vi "I2C_read.vi"(10 "错误输入（无错误）":errorcluster) -> (0 "readSucess":bool, 1 "buf":u8[](array[numeric]), 2 "Led":string, 3 "错误输出":errorcluster)   [LabVIEW 2017]
uses:
  jtool.dll
panel:
  out "reg_addr":u32
  out "slave_addr":u8
  out "init":string
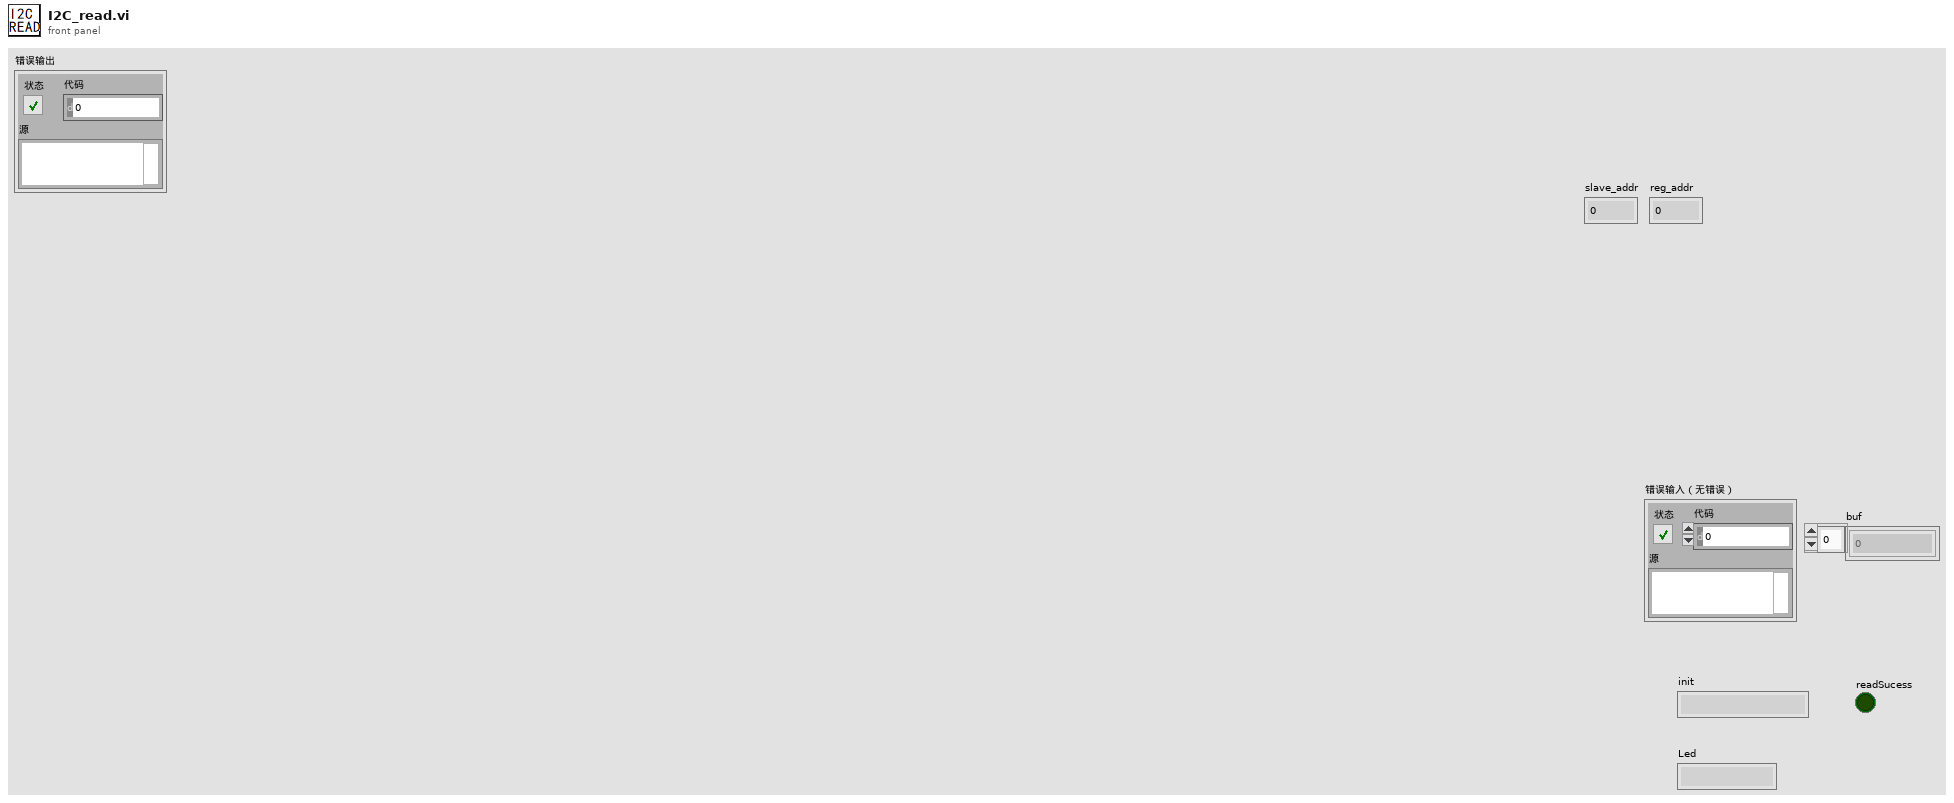
[diagram p1: front panel]
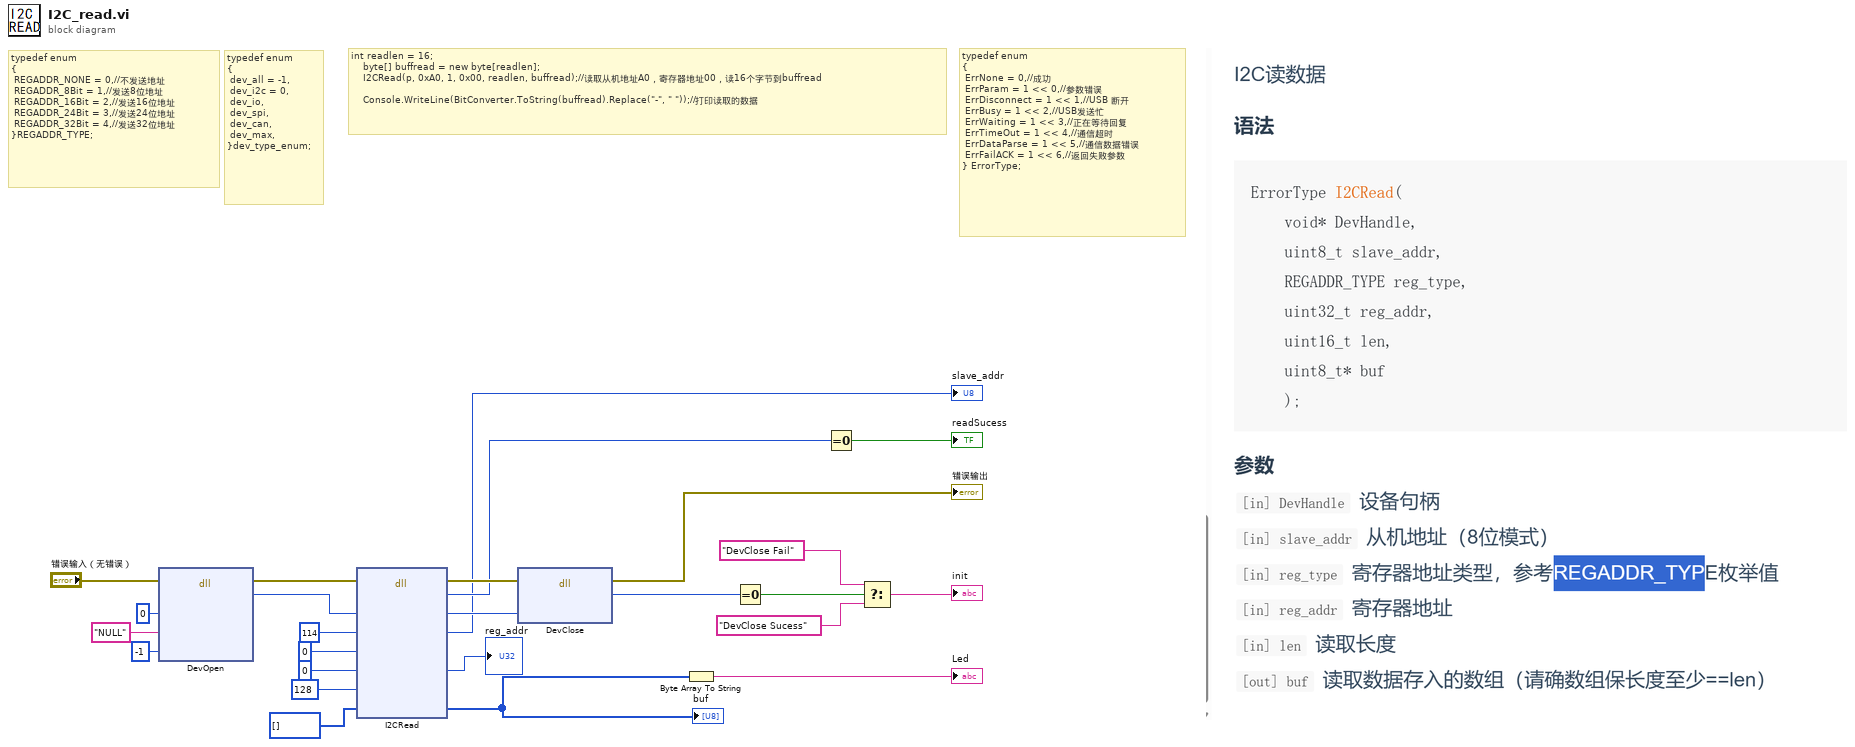
[diagram p0: block diagram]
diagram:
  # "typedef enum\n{\n\tErrNone = 0,//成功\n\tErrParam = 1 << 0,//参数错误\n\tErrDisconnect = 1 << 1,//USB 断开\n\tErrBusy = 1 << 2,//USB发送忙\n\tErrWaiting = 1 << 3,//正在等待回复\n\tErrTimeOut = 1 << 4,//通信超时\n\tErrDataParse = 1 << 5,//通信数据错误\n\tErrFailACK = 1 << 6,//返回失败参数\n} ErrorType;"
  # "typedef enum\n{\n\tdev_all = -1,\n\tdev_i2c = 0,\n\tdev_io,\n\tdev_spi,\n\tdev_can,\n\tdev_max,\n}dev_type_enum;"
  # "typedef enum\n{\n\tREGADDR_NONE = 0,//不发送地址\n\tREGADDR_8Bit = 1,//发送8位地址\n\tREGADDR_16Bit = 2,//发送16位地址\n\tREGADDR_24Bit = 3,//发送24位地址\n\tREGADDR_32Bit = 4,//发送32位地址\n}REGADDR_TYPE;"
  # "int readlen = 16;\n    byte[] buffread = new byte[readlen];\n    I2CRead(p, 0xA0, 1, 0x00, readlen, buffread);//读取从机地址A0，寄存器地址00，读16个字节到buffread\n\n    Console.WriteLine(BitConverter.ToString(buffread).Replace(\"-\", \" \"));//打印读取的数据"
  n1 = dll-call lib="D:/X682 Camera Calibration Tester Program/HardWare/Led_I2C2561/jtool.dll" fn="DevOpen"(error in="错误输入（无错误）", "DevType"=0, "Sn"="NULL", "Id"=-1) -> (error out=w9:errorcluster, "返回类型"=w8:i32)  [unwired: 5 in, 1 out]
  n2 = dll-call lib="D:/X682 Camera Calibration Tester Program/HardWare/Led_I2C2561/jtool.dll" fn="I2CRead"(error in=w9, "DevHandle"=w8, "slave_addr"=u8 114, "reg_type"=u8 0, "reg_addr"=u32 0, "len"=u16 128, "buf"=u8[] []) -> (error out=w11:errorcluster, "返回类型"=w6:u8, "DevHandle"=w10:i32, "slave_addr"=→"slave_addr":u8, "reg_addr"=→"reg_addr":u32, "buf"=w1:u8[])  [unwired: 4 in, 1 out]
  "buf" <- w1
  n3 = dll-call lib="D:/X682 Camera Calibration Tester Program/HardWare/Led_I2C2561/jtool.dll" fn="DevClose"(error in=w11, "DevHandle"=w10) -> (error out=→"错误输出":errorcluster, "返回类型"=w21:u8)  [unwired: 3 in, 1 out]
  n4 = Byte Array To String(unsigned byte array=w1) -> (string=→"Led":string)
  n5 = Equal To 0?(x=w21) -> (x = 0?=w20:bool)
  n6 = Equal To 0?(x=w6) -> (x = 0?=→"readSucess":bool)
  n7 = Select(t="DevClose Fail", s=w20, f="DevClose Sucess") -> (s? t:f=→"init":string)
